vi "GUI_HTT_BeamNetUS_HOFI.vi"() -> ()   [LabVIEW 2020]
uses:
  Shared/GUI_Template/GUI_master/tcp_new_data_event.ctl
  Shared/GUI_Template/GUI_master/tcp new data cluster.ctl
  GUI_TestStand/Fire button.ctl
panel:
  in  "Tab Control 3":enum32{"Pointing"}(tab)
  in  "Position.Axis 321::20":dbl caption="HoleyMirror X" min=-9999999999.0 max=9999999999.0
  in  "Position.Axis 322::20":dbl caption="HoleyMirror Y" min=-999999.0 max=999999.0
  in  "Position.Axis 311::20":dbl caption="ScatterIn X" min=-999999.0 max=999999.0
  in  "Position.Axis 312::20":dbl caption="ScatterIn Y" min=-999999.0 max=999999.0
  in  "Front_BackScatter":bool
  out "ProbeToScatter (ns)":dbl format="%#_4g"
  out "Scatter Delay (ns)":dbl format="%#_4g"
  out "Probe Delay (ns)":dbl format="%#_4g"
  in  "value5::19":dbl caption="Drive t0 (P short)" min=-9999999.0 max=9999999.0 format="%#_13g"
  out "pressure::28":dbl caption="Measured\nPressure" min=-100.0 max=500.0 format="%#_13g"
  in  "GUIdevice 28":string="HTT-Baratron"
  in  "GUIdevice 27":string="HTT_LowPressureControl"
  in  "GUIdevice 26":string="HTT-HOFI_GasCellLength"
  in  "pressure::27":dbl caption="Set Pressure" min=0.0 max=500.0 format="%#_13g"
  in  "position::26":dbl caption="Length" min=0.0 max=104.0 format="%#_13g"
  in  "GUIdevice 25":string="HTT-Hexapod"
  out "ypos::25":dbl caption="ypos (longitudinal)" min=-22.0 max=22.0 format="%#_13g"
  out "zpos::25":dbl caption="zpos (vertical)" min=-10.0 max=10.0 format="%#_13g"
  in  "xpos::25":dbl caption="xpos (left/right)" min=-25.0 max=25.0 format="%#_13g"
  in  "Position.Axis 112::24":dbl caption="Scatter Comp. Y" min=-999999.0 max=999999.0
  in  "Position.Axis 111::24":dbl caption="Scatter Comp. X" min=-999999.0 max=999999.0
  in  "Position.Axis 522::24":dbl caption="TC_In_y" min=-999999.0 max=999999.0
  in  "Position.Axis 521::24":dbl caption="TC_In_x" min=-999999.0 max=999999.0
  in  "GUIdevice 19":string="HTT-Manual_Parameter"
  in  "value9::19":dbl caption="Scatter t0 (S)" min=-9999999.0 max=9999999.0 format="%#_13g"
  in  "value8::19":dbl caption="Scatter t0 (P long)" min=-9999999.0 max=9999999.0 format="%#_13g"
  in  "value6::19":dbl caption="Drive t0 (P long)" min=-9999999.0 max=9999999.0 format="%#_13g"
  in  "value7::19":dbl caption="Scatter t0 (P short)" min=-9999999.0 max=9999999.0 format="%#_13g"
  in  "Position.Axis 3::10":dbl caption="Drive Ghost Stage" min=0.0 max=50.0
  in  "Position.Axis 342::20":dbl caption="GhostY" min=-999999.0 max=999999.0
  in  "Position.Axis 341::20":dbl caption="GhostX" min=-999999.0 max=999999.0
  in  "Position.Axis 1::15":dbl caption="S stage" min=-600.0 max=600.0
  in  "position::23":dbl caption="P LongStage" min=0.0 max=610.0
  in  "Position.Axis 3::6":dbl caption="P ShortStage" min=0.0 max=200.0
  in  "GUIdevice 24":string="HTT-PicoPad_LCave"
  in  "Tab Control 2":enum32{"Longitudinal", "Transverse"}(tab)
  in  "Position.Axis 433::20":dbl caption="FFy (Chamber)" min=-999999.0 max=999999.0
  in  "Position.Axis 431::20":dbl caption="FFx (Chamber)" min=-999999.0 max=999999.0
  in  "Position.Axis 322::24":dbl caption="probe_y (L-Cave)" min=-999999.0 max=999999.0
  in  "Position.Axis 321::24":dbl caption="probe_x (L-Cave)" min=-999999.0 max=999999.0
  in  "Position.Axis 112::20":dbl caption="Probe_TC_InY" min=-999999.0 max=999999.0
  in  "Position.Axis 111::20":dbl caption="Probe_TC_InX" min=-999999.0 max=999999.0
  in  "GUIdevice 23":string="HTT_ProbeLongDelay"
  in  "GUIdevice 22":string="Assert-Ctrl_DUTStage"
  in  "GUIdevice 21":string="HTT-LPModeStage"
  in  "Position.Ch6::22":dbl caption="Back Ceramic" min=0.0 max=200.0
  in  "position::21":dbl caption="LP Mode Imager" min=0.0 max=400.0
  in  "Position.Axis 432::20":dbl caption="Axicon Pitch (y)" min=-999999.0 max=999999.0
  in  "Position.Axis 341::20":dbl caption="Axicon Yaw (x)" min=-999999.0 max=999999.0
  in  "Position.Axis 2::3":dbl caption="Axicon stage y" min=0.0 max=25.0
  in  "Position.Axis 1::3":dbl caption="Axicon stage x" min=0.0 max=25.0
  in  "Tab Control":enum32{"OAP", "Pointing"}(tab)
  in  "Position.Axis 142::20":dbl caption="OutY" min=-999999.0 max=999999.0
  in  "Position.Axis 141::20":dbl caption="OutX" min=-999999.0 max=999999.0
  in  "Position.Axis 132::20":dbl caption="OAPInY" min=-999999.0 max=999999.0
  in  "Position.Axis 131::20":dbl caption="OAPInX" min=-1e+19 max=9999999999999.0
  in  "Position.Axis 212::20":dbl caption="FFY" min=-999999.0 max=999999.0
  in  "Position.Axis 211::20":dbl caption="FFX" min=-999999.0 max=999999.0
  in  "Position.Axis 122::20":dbl caption="NFY" min=-999999.0 max=999999.0
  in  "Position.Axis 121::20":dbl caption="NFX" min=-999999.0 max=999999.0
  in  "GUIdevice 20":string="HTT-PicoPad_BCave"
  in  "GUIdevice 18":string="HTT-DG645_6_B"
  in  "GUIdevice 17":string="HTT-ManualParameterBool"
  in  "GUIdevice 16":string="HTT-DG645_5Hz"
  in  "GUIdevice 15":string="HTT-NewportXPS"
  out "fire::12":string="fire" caption="fire"
  in  "GUIdevice 14":string="HTT-Energy-S-G"
  in  "GUIdevice 13":string="HTT-Energy-D"
  in  "Position.Axis 2::11":dbl caption="Translation" min=-50.0 max=50.0
  in  "Position.Axis 3::11":dbl caption="Rotation G1" min=-360.0 max=360.0
  in  "Position.Axis 1::11":dbl caption="Rotation G2" min=-360.0 max=360.0
  in  "GUIdevice 12":string="HTT-DG645"
  out "Position.Axis3::2":dbl caption="Rotation G1" min=-180.0 max=180.0 format="%#_13g"
  out "Position.Axis2::2":dbl caption="Rotation G2" min=-180.0 max=180.0 format="%#_13g"
  in  "Position.Axis1::2":dbl caption="Translation" min=-60000.0 max=60000.0 format="%#_13g"
  in  "GUIdevice 11":string="HTT-ESP05"
  in  "GUIdevice 8":string="HTT-BNC"
  in  "GUIdevice 6":string="HTT-ESP04"
  in  "GUIdevice 5":string="HTT-ESP03"
  in  "Fire Button":T1=TRUE
  out "error IO 2":errorcluster
  out "fire::10":string
  out "tcp data event":T2
  in  "UDP error message":string
  in  "GUIdevice 7":string="HTT-Pulsar"
  in  "GUIdevice 2":string="HTT-Aerotech"
  in  "GUIdevice 10":string="HTT-ESP06"
  in  "GUIdevice 4":string="HTT-ESP02"
  in  "GUIdevice 1":string="HTT-MagTeslameter-DTM141"
  in  "GUIdevice 3":string="HTT-ESP01"
  in  "GUIdevice 9":string="HTT-HighPressureDAQ"
  in  "stop":bool
  # "Energy"
  # "CAP"
  # "BeamNetUS - HOFI"
  # "Drive"
  # "Probe"
  # "Pointing into TC"
  # "Alignment Stages"
  # "Target"
  # "Hexapod"
  # "Gas Cell"
  # "HOFI Compressor"
  # "HOFI line"
  # "Pointing into TC"
  # "Axicon"
  # "Timing"
  # "Drive Compressor"
  # "Stage Positions"
  # "Delays"
  # "Reference Measurements"
  # "v0.7   04/16/2021"
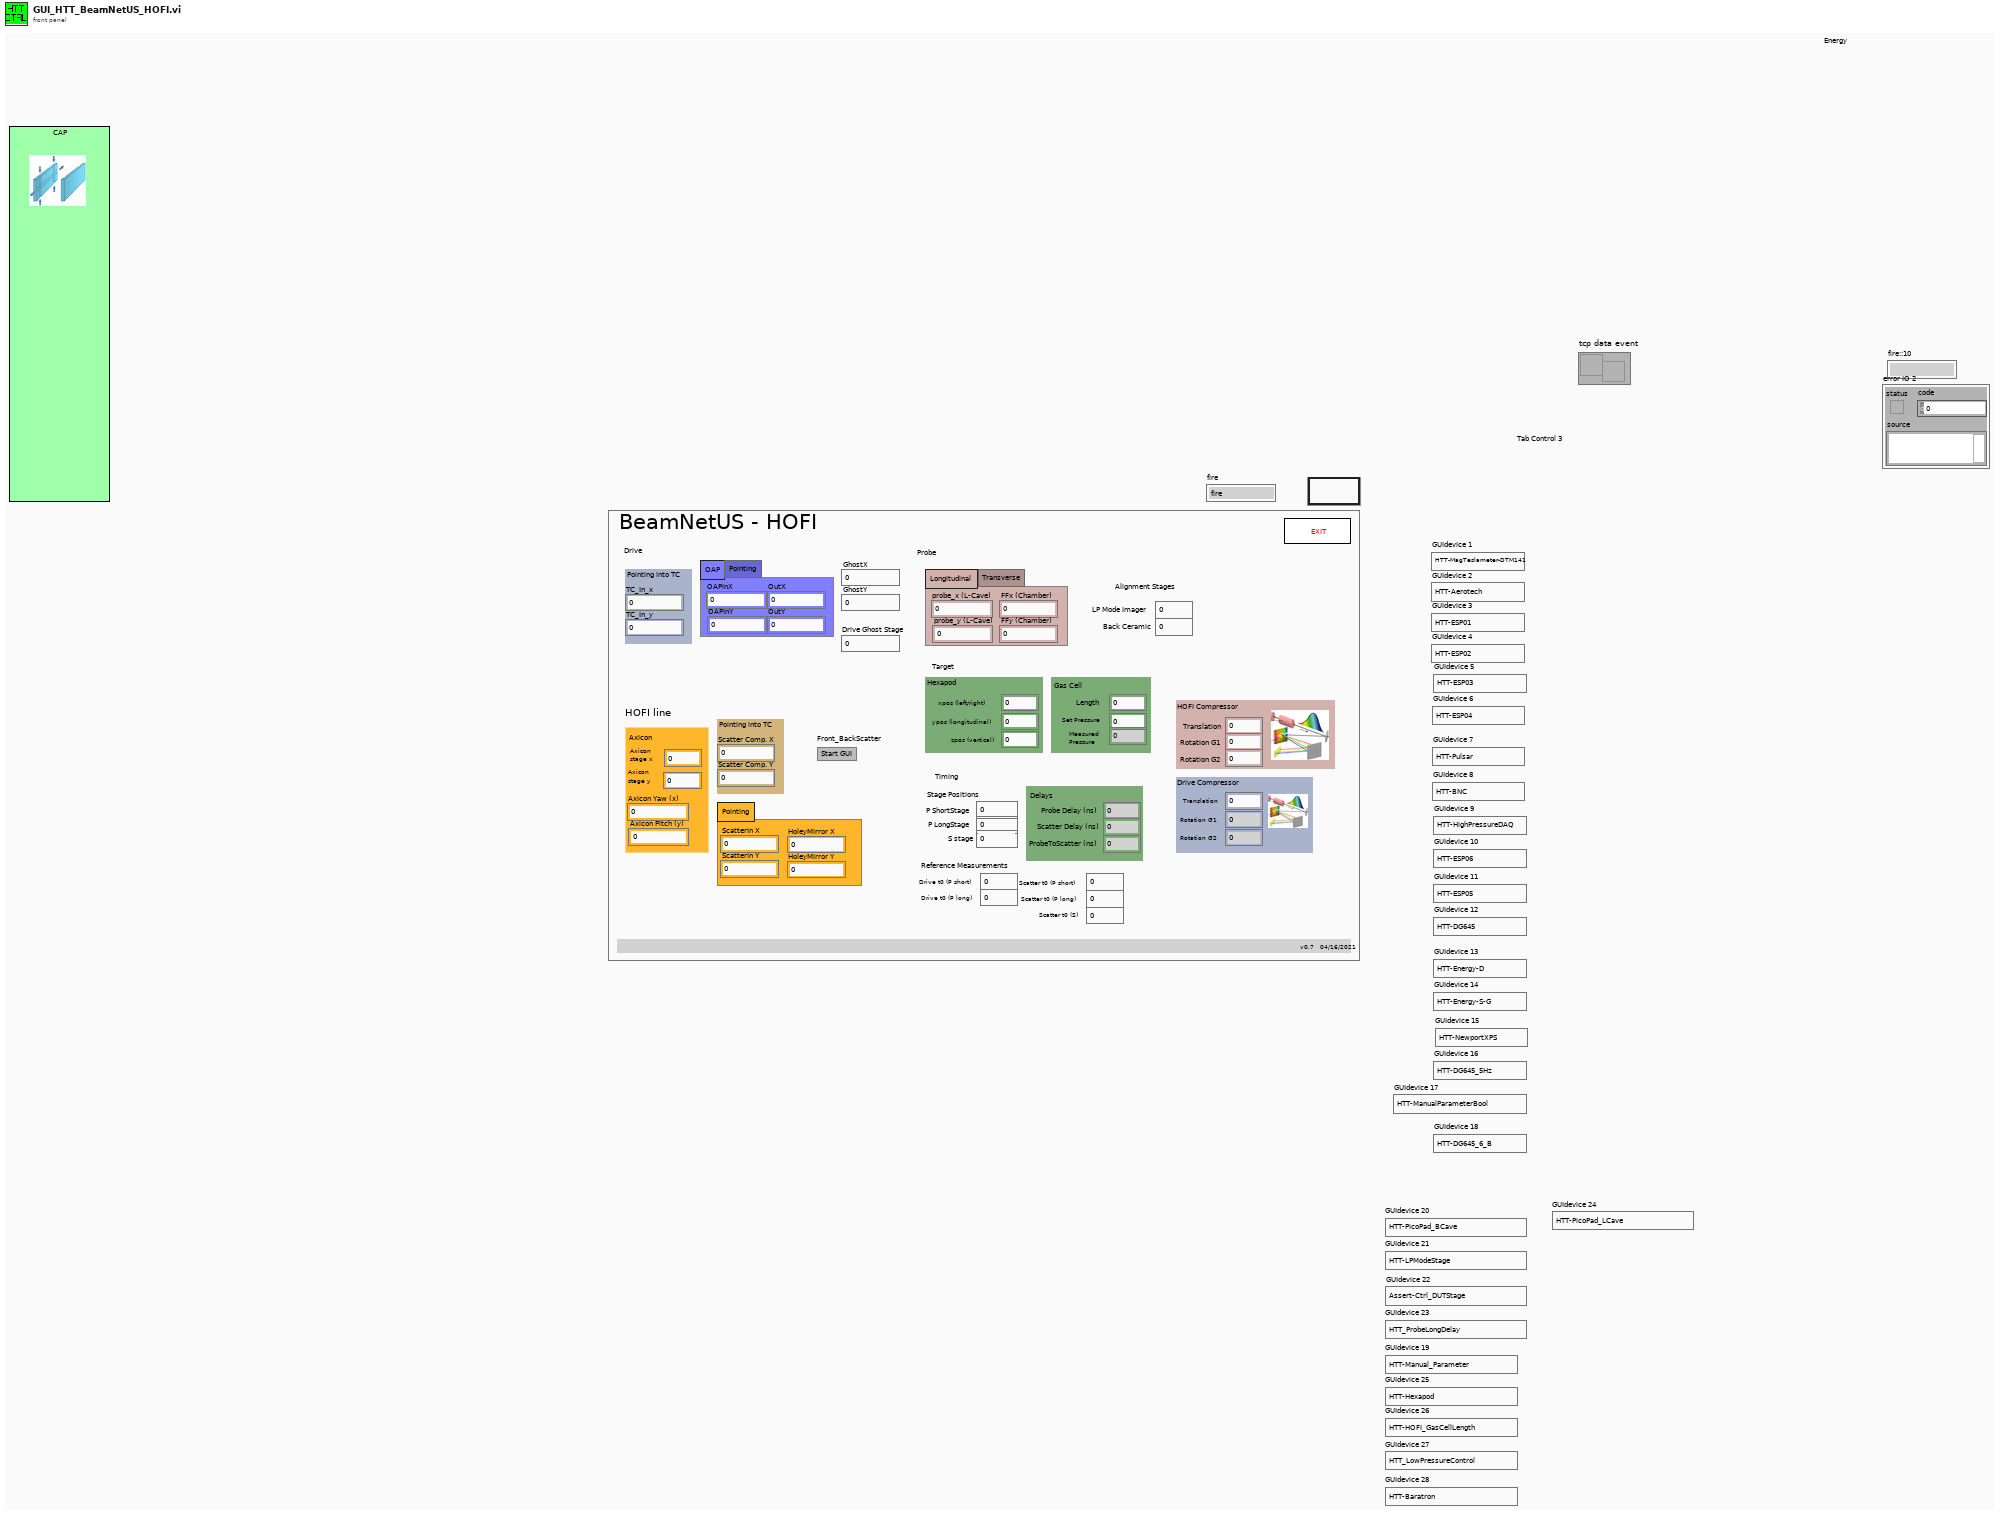
[diagram p1: front panel]
types:
  T1 = typedef "Fire button.ctl" = bool
  T2 = typedef "tcp_new_data_event.ctl" = refnum<user-event>
  T3 = typedef "tcp new data cluster.ctl" = cluster{"EventEnum":enum16{"new data", "connection status update"}, "Device name":string}
  T4 = enum32{"invalid app kind", "Development System", "Run Time System", "Student Edition", "Embedded LabVIEW", "Evaluation", "Custom"}
  T5 = enum32{"Invalid", "Standard", "Closed", "Hidden", "Minimized", "Maximized"}
  T6 = cluster{"Core":cluster{"Current VI Reference":refnum<vi>, "Close Panel on Exit?":bool}, "Heater timing offset":dbl, "Discharge timing offset":dbl, "Jet trigger":bool, "Tik1":u32, "Tik2":u32, "Fire Continues Allowed":bool, "Jet enable":bool}
  T7 = cluster{"Current VI Reference":refnum<vi>, "Close Panel on Exit?":bool}
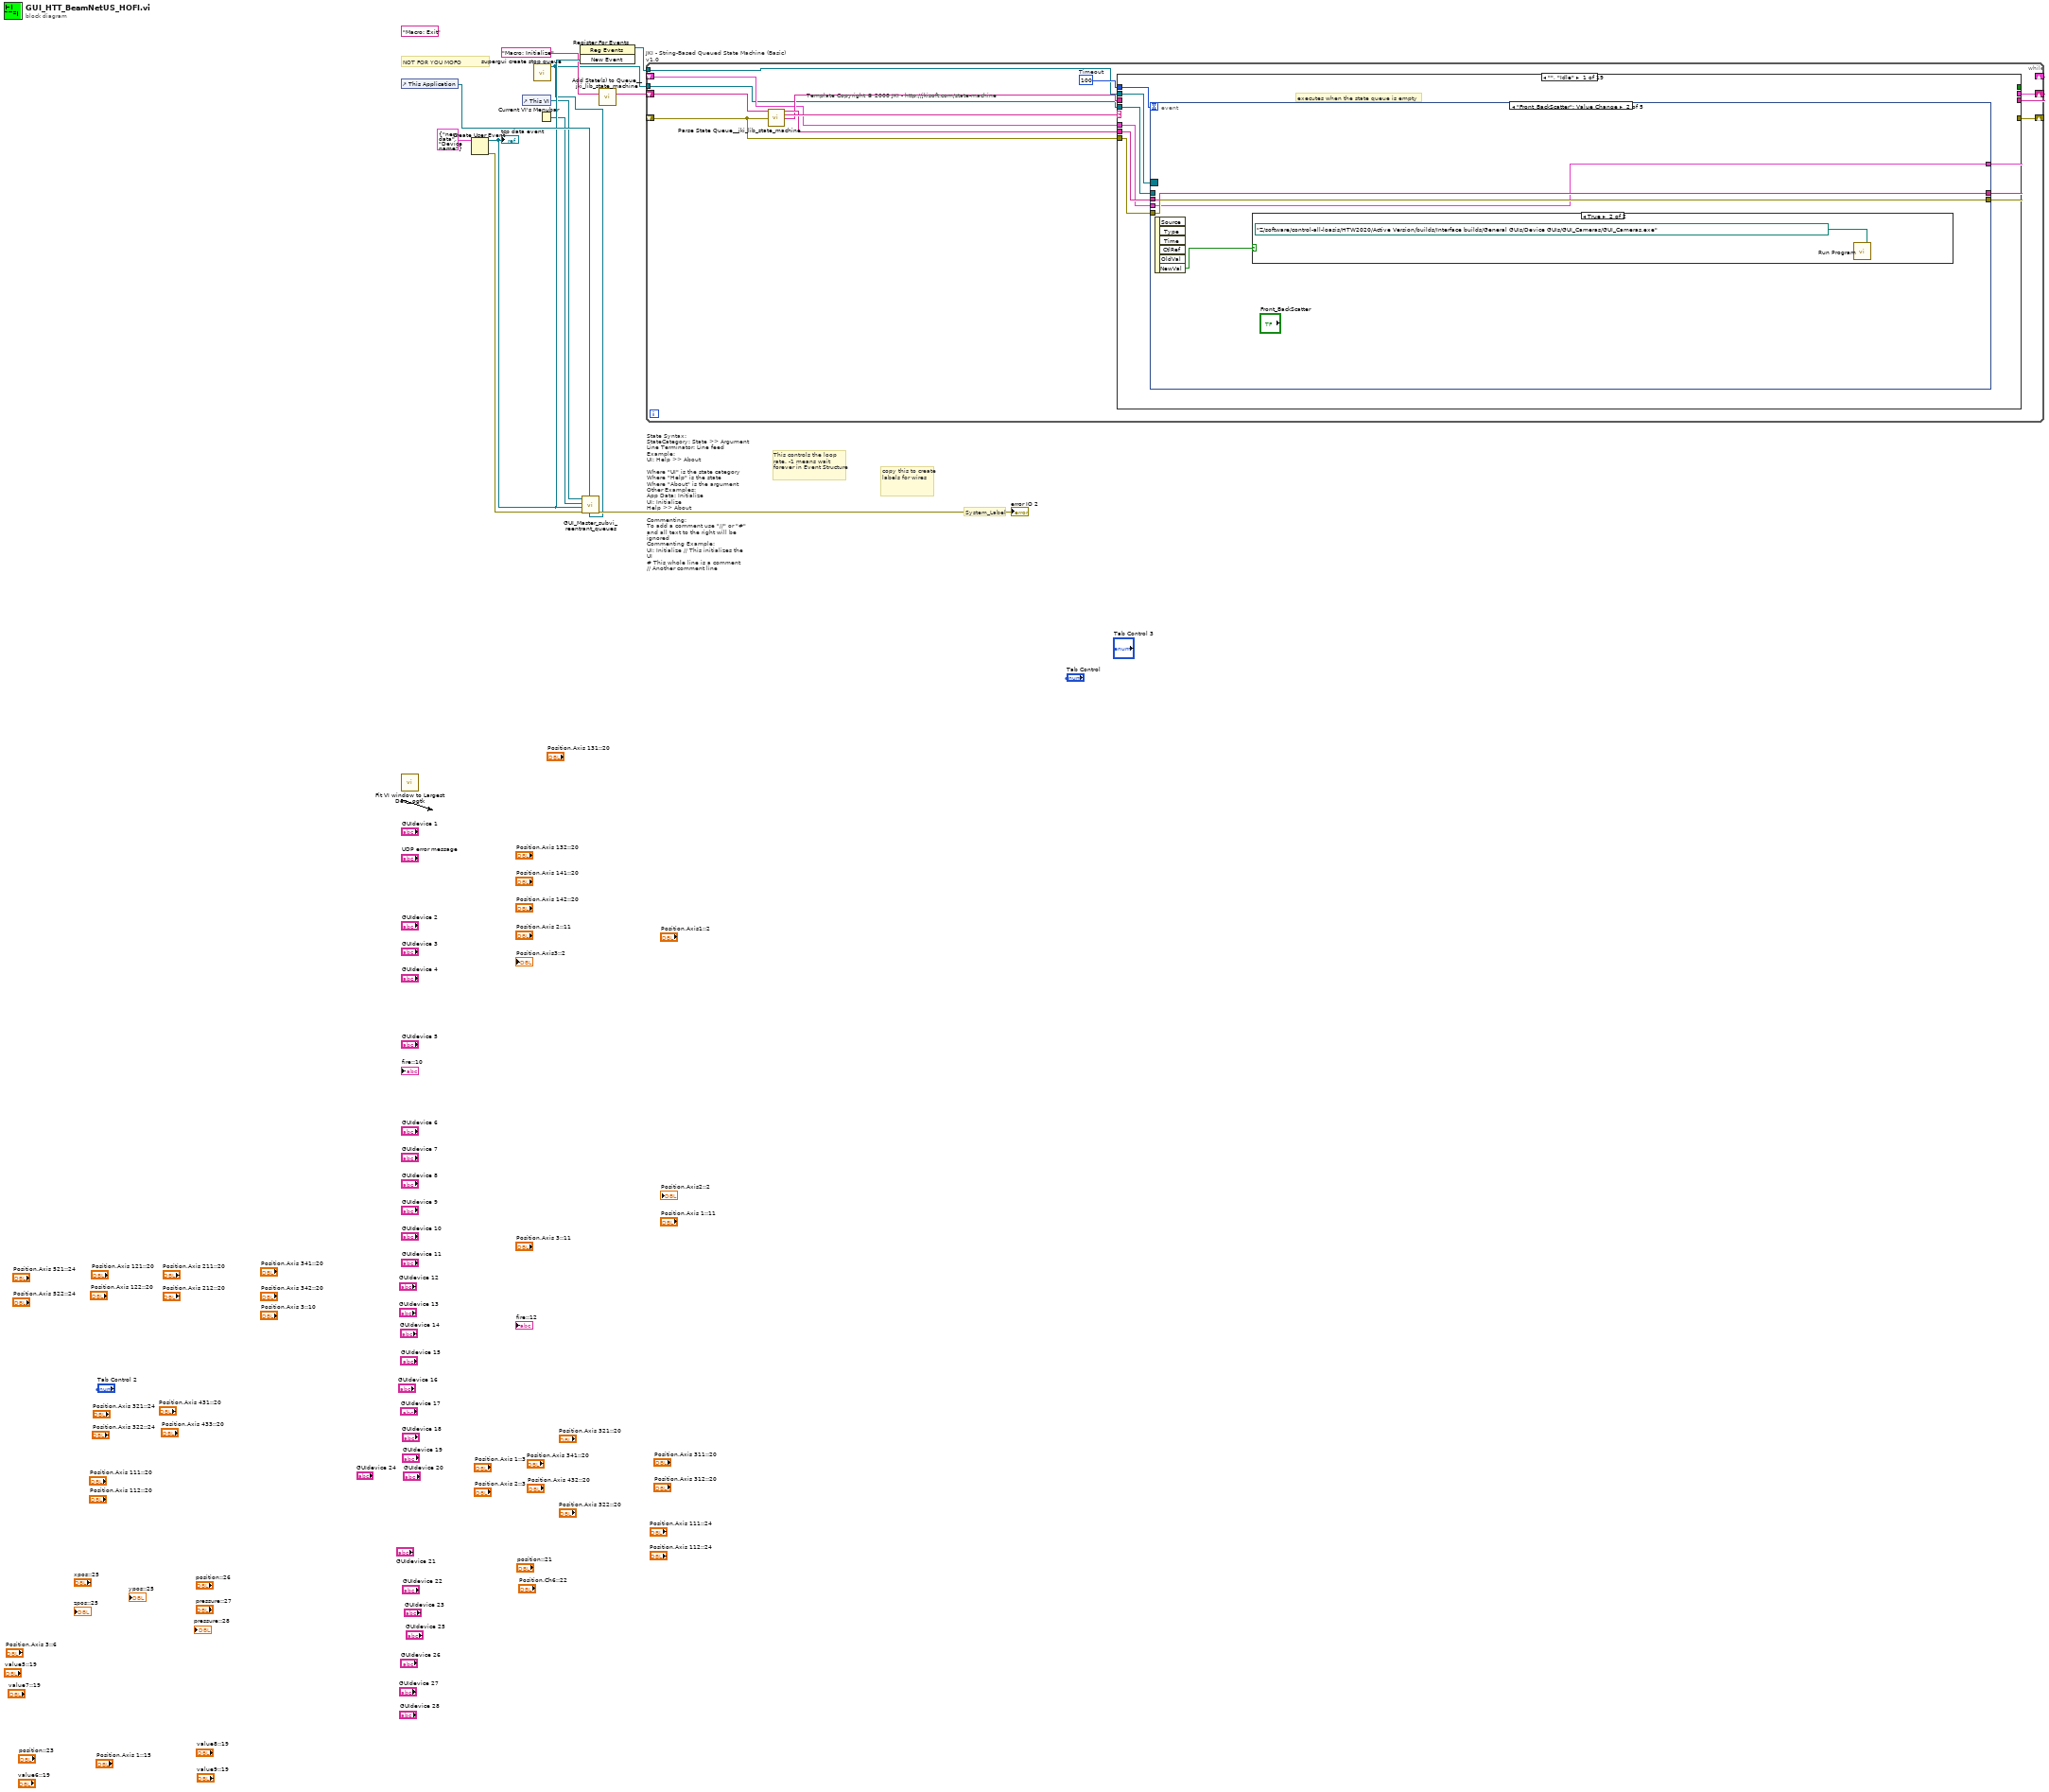
[diagram p0: block diagram]
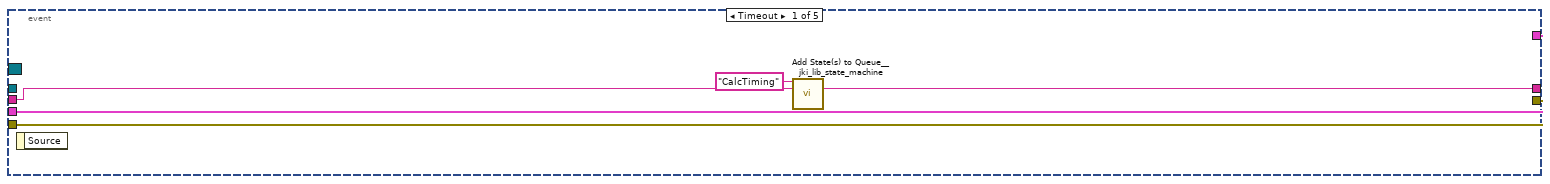
[diagram p2: hidden frame]
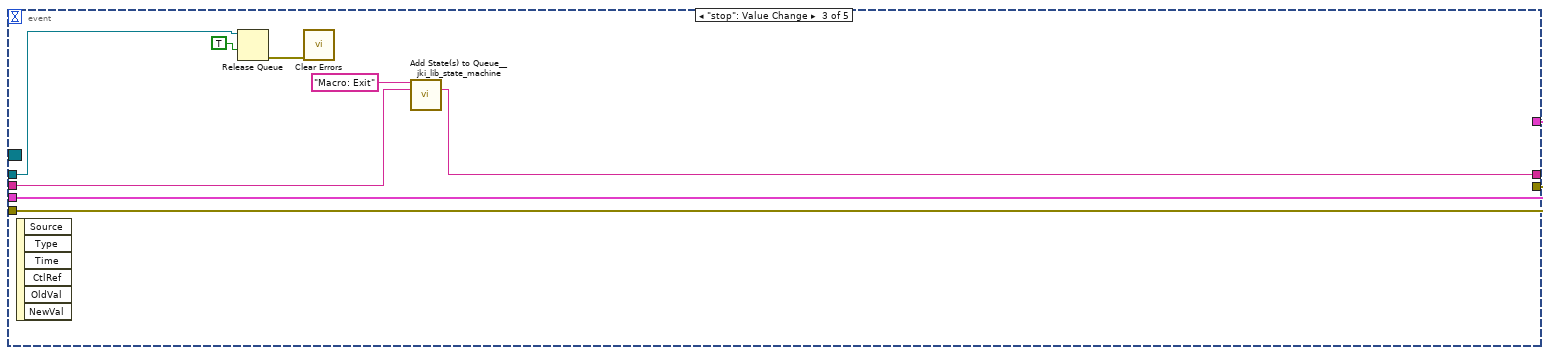
[diagram p4: hidden frame]
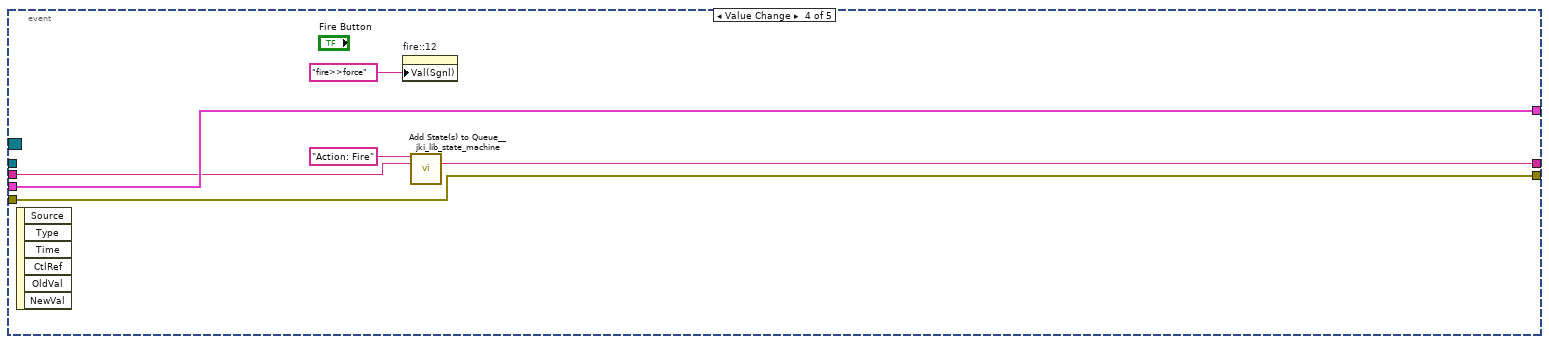
[diagram p5: hidden frame]
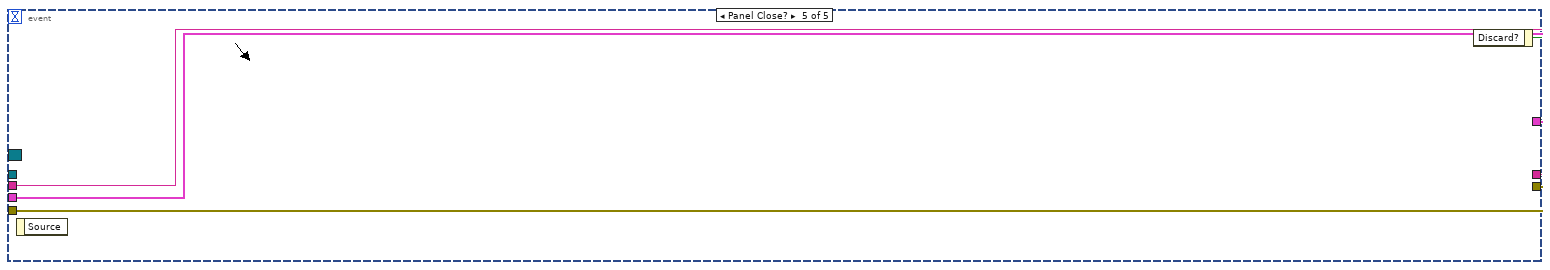
[diagram p6: hidden frame]
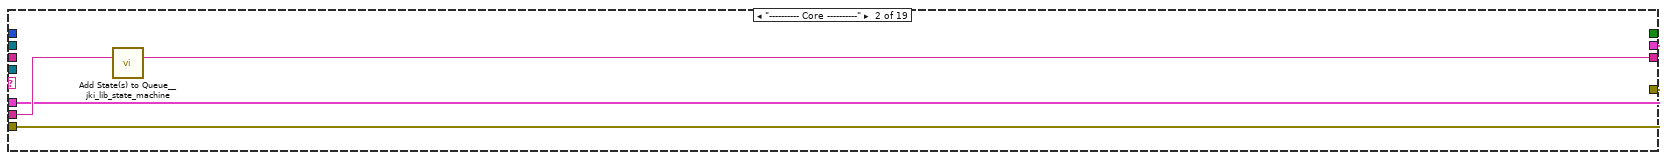
[diagram p7: hidden frame]
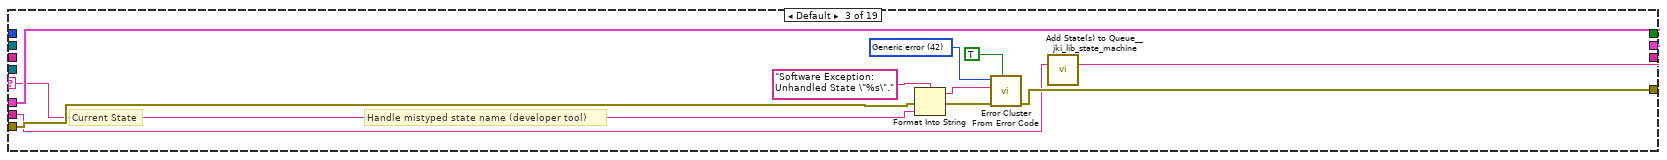
[diagram p8: hidden frame]
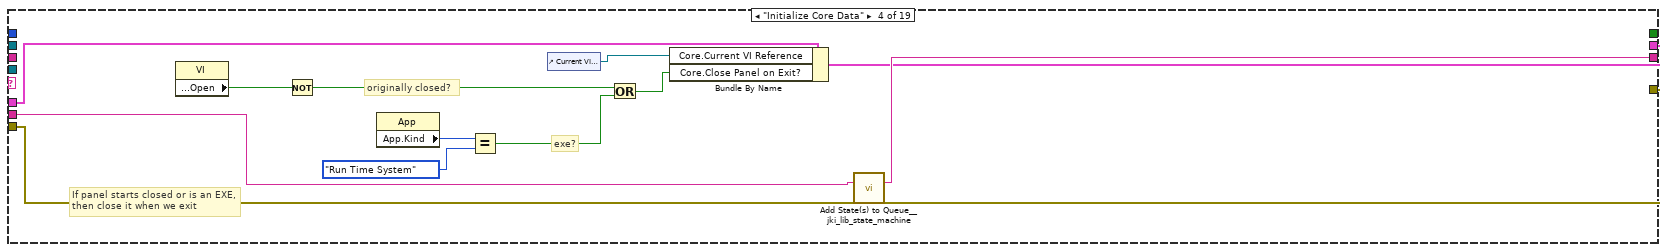
[diagram p9: hidden frame]
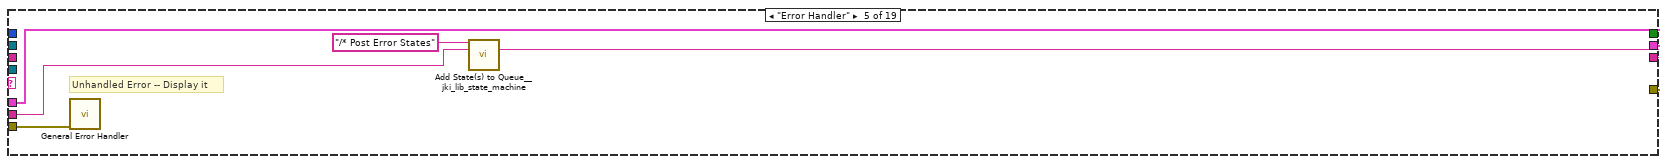
[diagram p10: hidden frame]
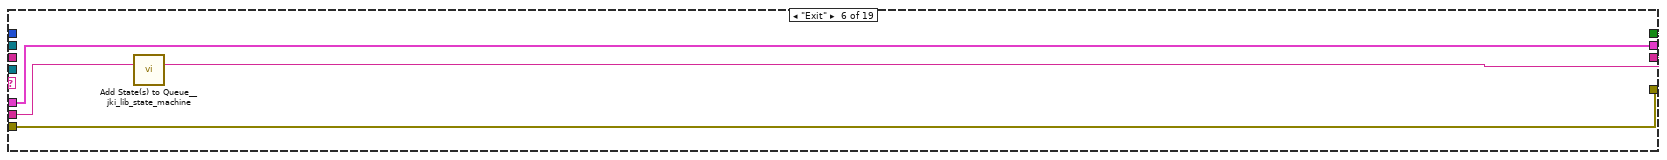
[diagram p11: hidden frame]
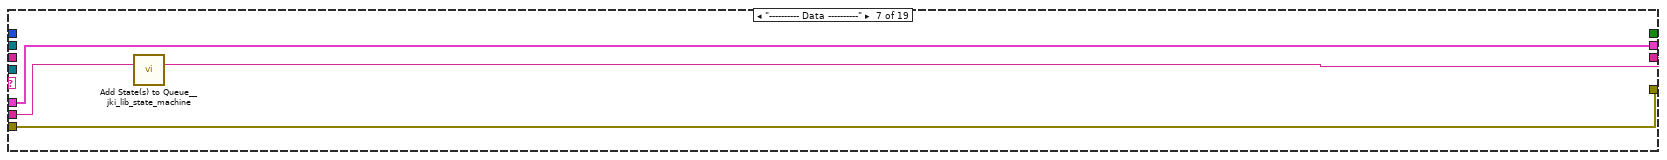
[diagram p12: hidden frame]
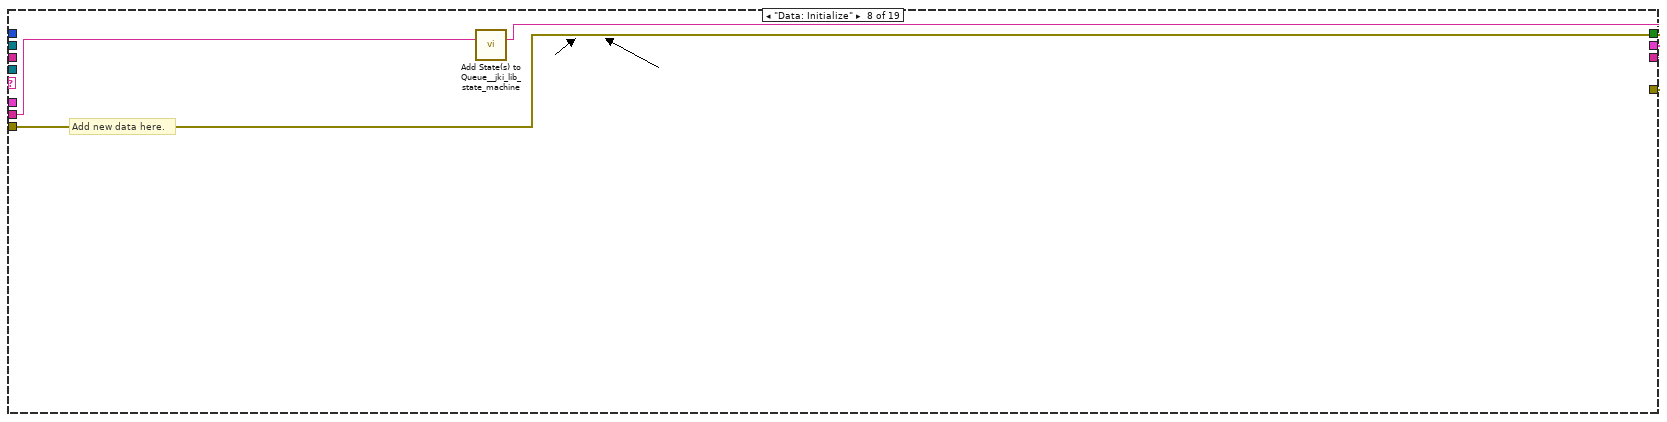
[diagram p13: hidden frame]
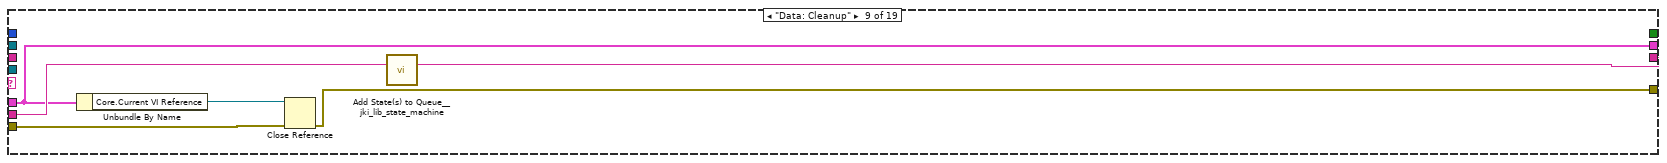
[diagram p14: hidden frame]
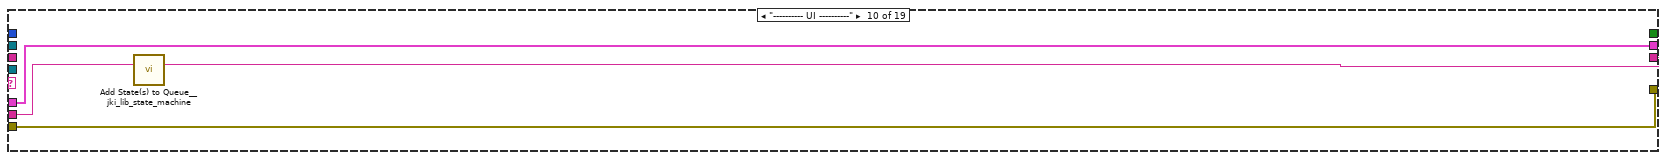
[diagram p15: hidden frame]
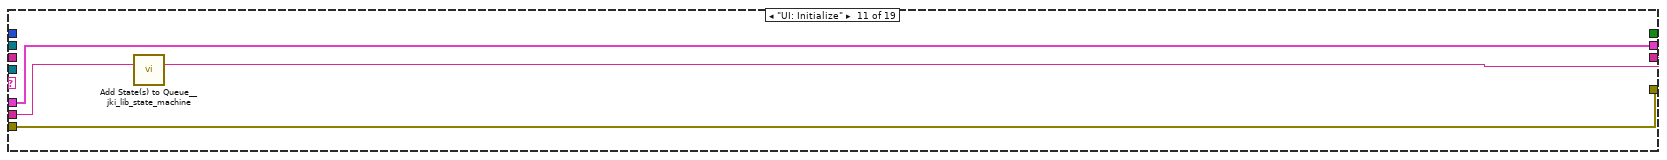
[diagram p16: hidden frame]
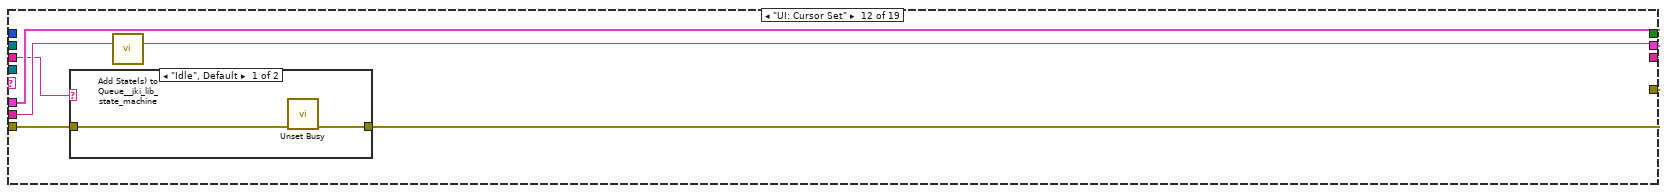
[diagram p17: hidden frame]
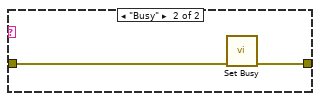
[diagram p18: hidden frame]
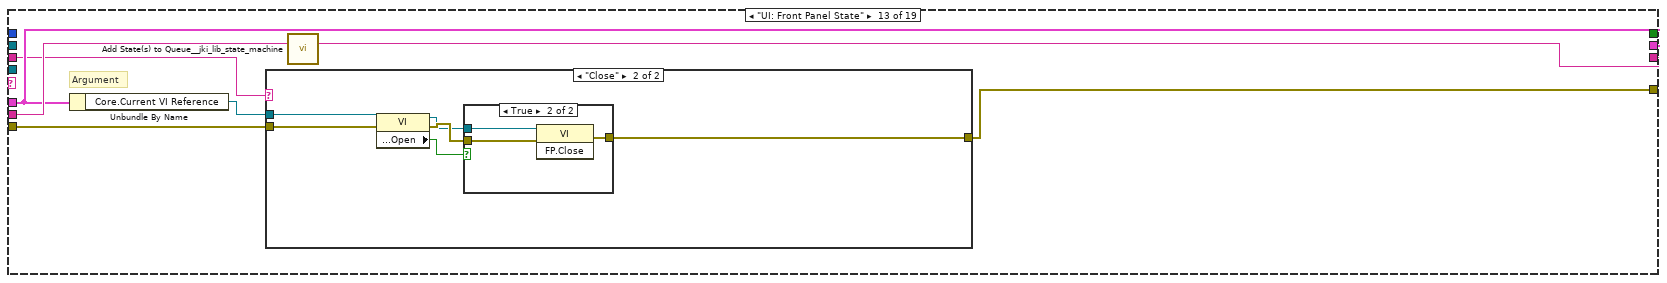
[diagram p19: hidden frame]
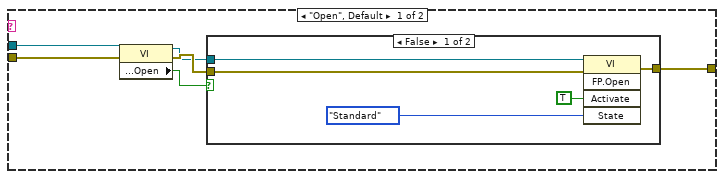
[diagram p20: hidden frame]
diagram:
  (unwired) "Macro: Exit"
  # "State Syntax:\nStateCategory: State >> Argument\nLine Terminator: Line feed\nExample:\nUI: Help >> About\n\nWhere \"UI\" is the state category\nWhere \"Help\" is the state\nWhere \"About\" is the argument\nOther Examples:\nApp Data: Initialize\nUI: Initialize\nHelp >> About\n\nCommenting:\nTo add a comment use \"//\" or \"#\" and all text to the right will be ignored\nCommenting Example:\nUI: Initialize // This initializes the UI\n# This whole line is a comment\n// Another comment line"
  # "copy this to create labels for wires"
  # "This controls the loop rate. -1 means wait forever in Event Structure"
  # "System_Label"
  # "NOT FOR YOU MOFO"
  n1 = control-ref of="This Application"() -> (w11:refnum<vi>)
  n2 = call <userlib>:"Fit VI window to Largest Dec__ogtk.vi"() -> ()  [unwired: 6 in, 2 out]
  n3 = Create User Event(user event datatype=T3 {"EventEnum"=enum."new data", "Device name"="Device name"} ("New Event")) -> (user event=w10:refnum<user-event>, error out=w9:errorcluster)  [unwired: 1 in]
  "tcp data event" <- w10
  n4 = control-ref of="This VI"() -> (w5:refnum<vi>)
  n5 = call "supergui create stop queue.vi"() -> ("STOP Queue out"=w2:refnum<queue>)  [unwired: 11 in]
  n6 = Current VI's Menubar() -> (w7:refnum<k9>)
  n7 = register-events(w10) -> (reference out=w1:refnum<event-registration>)  [unwired: 2 in, 1 out]
  n8 = call "GUI_Master_subvi_reentrant_queues.vi"("STOP Queue in"=w2, "This Application"=w11, "error in (no error)"=w9, "tcp data event"=w10, "Caller menu reference"=w7, "Caller VI ref"=w5) -> ("error out"=→"error IO 2":errorcluster)  [unwired: 5 in]
  n9 = call <vilib>:"Add State(s) to Queue__jki_lib_state_machine.vi"("State(s) in (\"\")"="Macro: Initialize") -> ("States Out"=w3:string)  [unwired: 14 in]
  n10 = while "JKI - String-Based Queued State Machine (Basic) v1.0" {
    shift-right: [w18] -> _
    shift-left: _ -> [w17]
    shift-right: [w20] -> _
    shift-left: _ -> [w15]
    shift-right: [w19] -> _
    shift-left: w3 -> [w21]
    tunnel: w1 -> [w14]
    tunnel: w2 -> [w13]
    stop <- w12 stop-if-true
    w16 = 100  # Timeout
    # "Template Copyright © 2008 JKI - http://jkisoft.com/state-machine"
    n11 = call <vilib>:"Parse State Queue__jki_lib_state_machine.vi"("State Queue"=w21, "Error In (no error)"=w15) -> ("Remaining States"=w23:string, "Current State"=w24:string, "Arguments"=w22:string)  [unwired: 11 in]
    n12 = case shown="\"\", \"Idle\"" w24 {
      selector: w24 -> [_ _ w68 _ _ _ _ _ _ _ _ _ _ _ _ _ _ _ _]
      tunnel: w23 -> [w33 w67 w72 w90 w96 w101 w105 w117 w123 w127 w131 w137 w148 w174 w211 w216 w226 w230 w236]
      tunnel: w22 -> [_ _ _ _ _ _ _ _ _ _ _ w132 w142 _ _ _ _ _ _]
      tunnel: w17 -> [w31 w64 w70 w81 w93 w99 w102 _ w118 w124 w129 w135 w144 w171 w208 w213 w223 w227 w234]
      tunnel: [w30 w65 w74 w87 errorcluster {"status"=FALSE, "code"=0, "source"=""} ("error out") w98 w103 w114 w119 w125 w128 w133 w145 w172 w209 w214 w224 w228 w231] -> w20
      tunnel: w15 -> [w29 w65 w73 w87 w92 w98 w103 w114 w120 w125 w128 w134 w146 w172 w209 w214 w224 w228 w232]
      tunnel: [w32 w66 w71 w89 w95 w100 w104 w116 w122 w126 w130 w136 w147 w173 w210 w215 w225 w229 w235] -> w19
      tunnel: [_ _ _ _ _ TRUE _ _ _ _ _ _ _ _ _ _ _ _ _] -> w12
      tunnel: [w25 w64 w70 w88 w93 w99 w102 w115 w118 w124 w129 w135 w144 w171 w208 w213 w223 w227 w234] -> w18
      tunnel: w16 -> [w28 _ _ _ _ _ _ _ _ _ _ _ _ _ _ _ _ _ _]
      tunnel: w14 -> [w27 _ _ _ _ _ _ _ _ _ _ _ _ _ _ _ _ _ _]
      tunnel: w13 -> [w26 _ _ _ _ _ _ _ _ _ _ _ _ _ _ _ _ _ _]
      frame "", "Idle" {
        # "executes when the state queue is empty"
        n13 = event shown="[1] \"Front_BackScatter\": Value Change" {
          selector: w27 -> [_ _ _ _ _]
          dyn-events: _ -> [_ _ _ _ _]
          timeout: w28 -> [_ _ _ _ _]
          tunnel: w33 -> [w38 w40 w51 w54 w63]
          tunnel: [w37 w40 w50 w55 w62] -> w32
          tunnel: w31 -> [w35 w39 w48 w57 w60]
          tunnel: [w36 w41 w49 w56 w61] -> w30
          tunnel: w29 -> [w36 w41 w49 w56 w61]
          tunnel: [w35 w39 w48 w57 w60] -> w25
          tunnel: w26 -> [_ _ w45 _ _]
          event Timeout {
            n14 = event-data() -> ()  [unwired: 1 in, 1 out]
            n15 = call <vilib>:"Add State(s) to Queue__jki_lib_state_machine.vi"("State(s) in Front (\"\")"="CalcTiming" ("State(s) in Front (\"\")"), "State(s) in (\"\")"=w38) -> ("States Out"=w37:string)  [unwired: 13 in]
          }
          event "Front_BackScatter": Value Change {
            n16 = event-data() -> ("NewVal"=w42:bool)  [unwired: 1 in, 5 out]
            n17 = case shown="True" w42 {
              frame False {
              }
              frame True {
                n18 = call "Run Program.vi"("Program Path"=path "Z:/software/control-all-loasis/HTW2020/Active Version/builds/Interface builds/General GUIs/Device GUIs/GUI_Cameras/GUI_Cameras.exe") -> ()  [unwired: 1 in]
              }
            }
          }
          event "stop": Value Change {
            # "Exit Button Value Change (pressed) Event\n(this executes Macro: Exit to terminate the VI)"
            n19 = event-data() -> ()  [unwired: 1 in, 6 out]
            n20 = Release Queue(queue=w45, force destroy? (F)=TRUE) -> (error out=w46:errorcluster)  [unwired: 1 in, 2 out]
            n21 = call <vilib>:"Clear Errors.vi"("error in (no error)"=w46) -> ()  [unwired: 5 in, 2 out]
            n22 = call <vilib>:"Add State(s) to Queue__jki_lib_state_machine.vi"("State(s) in Front (\"\")"="Macro: Exit", "State(s) in (\"\")"=w51) -> ("States Out"=w50:string)  [unwired: 13 in]
          }
          event Value Change {
            n23 = event-data() -> ()  [unwired: 1 in, 6 out]
            n24 = property on="fire::12" class="Str"("Val(Sgnl)"="fire>>force" ("Value (Signaling)")) -> ()  [unwired: 2 in, 2 out]
            n25 = call <vilib>:"Add State(s) to Queue__jki_lib_state_machine.vi"("State(s) in Front (\"\")"="Action: Fire" ("State(s) in Front (\"\")"), "State(s) in (\"\")"=w54) -> ("States Out"=w55:string)  [unwired: 13 in]
          }
          event Panel Close? {
            # "Discard the event because we'll close the front panel ourselves in Macro: Exit"
            # "Close Panel button (pressed) Event\n(this executes Macro: Exit to terminate the VI)"
            n26 = event-data() -> ()  [unwired: 1 in, 1 out]
            n27 = event-data("Discard?"=TRUE) -> ()  [unwired: 1 in, 1 out]
            n28 = call <vilib>:"Add State(s) to Queue__jki_lib_state_machine.vi"("State(s) in Front (\"\")"="Macro: Exit", "State(s) in (\"\")"=w63) -> ("States Out"=w62:string)  [unwired: 13 in]
          }
        }
      }
      frame "---------- Core ----------" {
        # "Do not put any code in this frame.\n(it is a separator no-op)"
        n29 = call <vilib>:"Add State(s) to Queue__jki_lib_state_machine.vi"("State(s) in (\"\")"=w67) -> ("States Out"=w66:string)  [unwired: 14 in]
      }
      frame Default {
        w77 = 42 items=["No error", "Argument error", "Memory is full", "Out of zone", "End of file", "File already open", "Generic file I/O error", "File not found", "File permission error", "Disk is full", "Duplicate path", "Too many files open", "System feature not enabled", "Resource file not found", "Cannot add resource", "Resource not found", "Image not found", "Image memory error", "Pen does not exist", "Config type invalid", "Config token not found", "Config parse error", "Config memory error", "Bad external code format", "Bad external code offset", "External code not present", "Null window", "Destroy window error", "Null menu", "Print aborted", "Bad print record", "Print driver error", "Windows error during printing", "Memory error during printing", "Print dialog error", "Generic print error", "Invalid device refnum", "Device not found", "Device parameter error", "Device unit error", "Cannot open device", "Device call aborted", "Generic error", "Cancelled by user", "Object ID too low", "Object ID too high", "Object not in heap", "Unknown heap", "Unknown object (invalid DefProc)", "Unknown object (DefProc not in table)", "Message out of range", "Invalid (null) method", "Unknown message", "Manager call not supported", "Bad address", "Network operation in progress", "Network operation timed out", "Connection is busy", "Network attribute not supported", "Network error", "Address in use", "System out of memory", "Connection aborted", "Connection refused", "Not connected", "Already connected", "Connection closed", "Initialization error (interapplication manager)", "Bad occurrence", "Wait on unbound occurrence handler", "Occurrence queue overflow", "Datalog type conflict", "Unused", "Unrecognized type (interapplication manager)", "Memory corrupt", "Failed to make temporary DLL", "Old CIN version", "Drag socket not found", "Failed to load drop-object", "Failed to register OLE object", "Failed to release OLE object", "Format specifier type mismatch", "Unknown format specifier", "Too few format specifiers", "Too many format specifiers", "Scan failed", "Newer CIN version", "Error converting to variant", "Runtime menu error", "Password tampered", "Variant attribute not found", "Incompatible variant data type", "Event data is not available", "Event Store is not present", "Occurrence is not found", "Event Queue is not created", "Event info is not available", "Refnum passed is NULL", "Error retrieving Class GUID", "Error retrieving CoClass GUID", "Error retrieving TypeLib GUID.", "Bad built application magic bytes.", "Specific driver is different from the specific driver associated with the Logical Name.", "There is no session opened to the class driver.", "Max Error", "MAX - Error with config objects", "MAX - Error loading configuration", "MAX - Group not supported"]
        # "Current State"
        # "Do not delete, rename, or modify this frame.\n(this is used to capture unhandled states and typos)"
        # "Handle mistyped state name (developer tool)"
        n30 = Format Into String(format string="Software Exception: Unhandled State \"%s\"." ("message"), error in=w73, w68) -> (resulting string=w76:string, error out=w75:errorcluster)  [unwired: 1 in]
        n31 = call <vilib>:"Error Cluster From Error Code.vi"("show call chain? (False)"=TRUE, "error in (no error)"=w75, "error message (\"\")"=w76, "error code (0)"=w77) -> ("error out"=w74:errorcluster)  [unwired: 5 in]
        n32 = call <vilib>:"Add State(s) to Queue__jki_lib_state_machine.vi"("State(s) in (\"\")"=w72) -> ("States Out"=w71:string)  [unwired: 14 in]
      }
      frame "Initialize Core Data" {
        # "Do not delete, rename, or modify this frame.\n(this is used to determine panel behavior on exit)"
        # "originally closed?"
        # "exe?"
        # "If panel starts closed or is an EXE, then close it when we exit"
        n33 = property class="VI"() -> ("Front Panel.Open"=w86:bool)  [unwired: 2 in, 2 out]
        n34 = Not(x=w86) -> (.not. x?=w83:bool)
        n35 = property class="App"() -> ("App.Kind"=w85:T4)  [unwired: 2 in, 2 out]
        n36 = Equal?(x=w85, y=T4."Run Time System" ("Application:Kind")) -> (x = y?=w82:bool)
        n37 = control-ref of="Current VI Reference"() -> (w79:refnum<vi>)
        n38 = Or(x=w83, y=w82) -> (x .or. y?=w80:bool)
        n39 = Bundle By Name(cluster=w81, "Core.Current VI Reference"=w79, "Core.Close Panel on Exit?"=w80) -> (w88:T6)
        n40 = call <vilib>:"Add State(s) to Queue__jki_lib_state_machine.vi"("State(s) in (\"\")"=w90) -> ("States Out"=w89:string)  [unwired: 14 in]
      }
      frame "Error Handler" {
        # "Unhandled Error -- Display it"
        # "Handle any errors here.\nYou can also output any states to clean-up after errors occur"
        # "Clear error"
        n41 = call <vilib>:"General Error Handler.vi"("error in (no error)"=w92) -> ()  [unwired: 10 in, 5 out]
        n42 = call <vilib>:"Add State(s) to Queue__jki_lib_state_machine.vi"("State(s) in Front (\"\")"="/* Post Error States", "State(s) in (\"\")"=w96) -> ("States Out"=w95:string)  [unwired: 13 in]
      }
      frame "Exit" {
        # "Do not put any code in this frame.\n(No errors that occur here will be handled.)"
        n43 = call <vilib>:"Add State(s) to Queue__jki_lib_state_machine.vi"("State(s) in (\"\")"=w101) -> ("States Out"=w100:string)  [unwired: 14 in]
      }
      frame "---------- Data ----------" {
        # "Do not put any code in this frame.\n(It is a separator no-op. You can make a copy of this frame to create a new Data frame)"
        n44 = call <vilib>:"Add State(s) to Queue__jki_lib_state_machine.vi"("State(s) in (\"\")"=w105) -> ("States Out"=w104:string)  [unwired: 14 in]
      }
      frame "Data: Initialize" {
        w106 = FALSE  # Jet enable
        w107 = FALSE  # Fire Continues Allowed
        w109 = u32 0  # Tik1
        w108 = u32 0  # Tik2
        w110 = FALSE  # Jet trigger
        w111 = 0.0  # Discharge timing offset
        w112 = 0.0  # Heater timing offset
        w113 = T7 {"Current VI Reference"=refnum, "Close Panel on Exit?"=FALSE}  # Core
        # "do not delete - used by framework"
        # "Expand Bundle to add new data elements to shift register data."
        # "Add new data here."
        # "Data names and types of shift register data are defined by this bundle."
        # "Initialize the shift-register data, here.\n(data names are defined by what you wire into the bundle function)"
        n45 = call <vilib>:"Add State(s) to Queue__jki_lib_state_machine.vi"("State(s) in (\"\")"=w117) -> ("States Out"=w116:string)  [unwired: 14 in]
        n46 = Bundle("Core"=w113, "Heater timing offset"=w112, "Discharge timing offset"=w111, "Jet trigger"=w110, "Tik1"=w109, "Tik2"=w108, "Fire Continues Allowed"=w107, "Jet enable"=w106) -> (w115:T6)  [unwired: 1 in]
      }
      frame "Data: Cleanup" {
        # "Cleanup any data and references, here.\n(this is called automatically, by the Macro: Exit)"
        n47 = Unbundle By Name(w118) -> ("Core.Current VI Reference"=w121:refnum<vi>)
        n48 = Close Reference(reference=w121, error in (no error)=w120) -> (error out=w119:errorcluster)
        n49 = call <vilib>:"Add State(s) to Queue__jki_lib_state_machine.vi"("State(s) in (\"\")"=w123) -> ("States Out"=w122:string)  [unwired: 14 in]
      }
      frame "---------- UI ----------" {
        # "Do not put any code in this frame.\n(It is a separator no-op. You can make a copy of this frame to create a new UI frame)"
        n50 = call <vilib>:"Add State(s) to Queue__jki_lib_state_machine.vi"("State(s) in (\"\")"=w127) -> ("States Out"=w126:string)  [unwired: 14 in]
      }
      frame "UI: Initialize" {
        # "Initialize the User Interface, here.\n(this is called automatically, by the Macro: Init)"
        n51 = call <vilib>:"Add State(s) to Queue__jki_lib_state_machine.vi"("State(s) in (\"\")"=w131) -> ("States Out"=w130:string)  [unwired: 14 in]
      }
      frame "UI: Cursor Set" {
        # "Argument"
        # "Set and Unset Cursor Busy.\n(Usage: \"UI: Cursor Set >> Busy|Idle\")"
        n52 = case shown="\"Idle\", Default" w132 {
          tunnel: w134 -> [w139 w141]
          tunnel: [w138 w140] -> w133
          frame "Idle", Default {
            n53 = call <vilib>:"Unset Busy.vi"("error in (no error)"=w139) -> ("error out"=w138:errorcluster)  [unwired: 10 in]
          }
          frame "Busy" {
            n54 = call <vilib>:"Set Busy.vi"("error in (no error)"=w141) -> ("error out"=w140:errorcluster)  [unwired: 9 in, 1 out]
          }
        }
        n55 = call <vilib>:"Add State(s) to Queue__jki_lib_state_machine.vi"("State(s) in (\"\")"=w137) -> ("States Out"=w136:string)  [unwired: 14 in]
      }
      frame "UI: Front Panel State" {
        # "Argument"
        # "Set Front Panel Open or Closed\n(Usage: \"UI: Front Panel State >> Open|Close\")"
        n56 = Unbundle By Name(w144) -> ("Core.Current VI Reference"=w143:refnum<vi>)
        n57 = case shown="\"Close\"" w142 {
          tunnel: w146 -> [w152 w165]
          tunnel: [w154 w166] -> w145
          tunnel: w143 -> [w153 w163]
          frame "Open", Default {
            n58 = property class="VI"(reference=w153, error in=w152) -> (reference out=w150:refnum<vi>, error out=w151:errorcluster, "Front Panel.Open"=w149:bool)
            n59 = case shown="False" w149 {
              tunnel: [w157 w160] -> w154
              tunnel: w151 -> [w156 w160]
              tunnel: w150 -> [w155 _]
              frame False {
                n60 = invoke class="VI" method="FP.Open"(reference=w155, error in=w156, "Activate"=TRUE, "State"=T5."Standard") -> (error out=w157:errorcluster)  [unwired: 1 in, 4 out]
              }
              frame True {
              }
            }
          }
          frame "Close" {
            n61 = property class="VI"(reference=w163, error in=w165) -> (reference out=w162:refnum<vi>, error out=w164:errorcluster, "Front Panel.Open"=w161:bool)
            n62 = case shown="True" w161 {
              tunnel: [w167 w170] -> w166
              tunnel: w164 -> [w167 w169]
              tunnel: w162 -> [_ w168]
              frame False {
              }
              frame True {
                n63 = invoke class="VI" method="FP.Close"(reference=w168, error in=w169) -> (error out=w170:errorcluster)  [unwired: 1 in, 2 out]
              }
            }
          }
        }
        n64 = call <vilib>:"Add State(s) to Queue__jki_lib_state_machine.vi"("State(s) in (\"\")"=w148) -> ("States Out"=w147:string)  [unwired: 14 in]
      }
      frame "---------- Macro ----------" {
        # "Do not put any code in this frame.\n(It is a separator no-op. You can make a copy of this frame to create a new Macro frame)"
        n65 = call <vilib>:"Add State(s) to Queue__jki_lib_state_machine.vi"("State(s) in (\"\")"=w174) -> ("States Out"=w173:string)  [unwired: 14 in]
      }
      frame "CalcTiming" {
        # "Do not put any code in this frame.\n(It is a separator no-op. You can make a copy of this frame to create a new Macro frame)"
        n66 = property on="value7::19" class="DigNum (strict)"() -> ("Value"=w182:dbl)  [unwired: 2 in, 2 out]
        n67 = property on="value5::19" class="DigNum (strict)"() -> ("Value"=w183:dbl)  [unwired: 2 in, 2 out]
        n68 = property on="value8::19" class="DigNum (strict)"() -> ("Value"=w188:dbl)  [unwired: 2 in, 2 out]
        n69 = property on="value6::19" class="DigNum (strict)"() -> ("Value"=w187:dbl)  [unwired: 2 in, 2 out]
        n70 = property on="Position.Axis 1::15" class="DigNum (strict)"() -> ("Value"=w189:dbl)  [unwired: 2 in, 2 out]
        n71 = property on="value9::19" class="DigNum (strict)"() -> ("Value"=w190:dbl)  [unwired: 2 in, 2 out]
        n72 = call <vilib>:"Add State(s) to Queue__jki_lib_state_machine.vi"("State(s) in (\"\")"=w211) -> ("States Out"=w210:string)  [unwired: 14 in]
        n73 = Subtract(x=w182, y=w183) -> (x-y=w184:dbl)
        n74 = Subtract(x=w188, y=w187) -> (x-y=w185:dbl)
        n75 = Subtract(x=w189, y=w190) -> (x-y=w186:dbl)
        n76 = Multiply(x=-2, y=w186) -> (x*y=w193:dbl)
        n77 = Multiply(x=-2, y=w184) -> (x*y=w191:dbl)
        n78 = Multiply(x=-4, y=w185) -> (x*y=w194:dbl)
        n79 = Add(x=w191, y=w194) -> (x+y=w192:dbl)
        n80 = Add(x=w192, y=w193) -> (x+y=w195:dbl)
        n81 = Divide(x=w195, y=300) -> (x/y=w175:dbl)
        "Scatter Delay (ns)" <- w175
        n82 = property on="Position.Axis 3::6" class="DigNum (strict)"() -> ("Value"=w204:dbl)  [unwired: 2 in, 2 out]
        n83 = property on="value6::19" class="DigNum (strict)"() -> ("Value"=w207:dbl)  [unwired: 2 in, 2 out]
        n84 = property on="value5::19" class="DigNum (strict)"() -> ("Value"=w205:dbl)  [unwired: 2 in, 2 out]
        n85 = property on="position::23" class="DigNum (strict)"() -> ("Value"=w206:dbl)  [unwired: 2 in, 2 out]
        n86 = Subtract(x=w204, y=w205) -> (x-y=w199:dbl)
        n87 = Subtract(x=w206, y=w207) -> (x-y=w200:dbl)
        n88 = Multiply(x=-2, y=w199) -> (x*y=w201:dbl)
        n89 = Multiply(x=-4, y=w200) -> (x*y=w202:dbl)
        n90 = Add(x=w201, y=w202) -> (x+y=w203:dbl)
        n91 = Divide(x=w203, y=300) -> (x/y=w176:dbl)
        "Probe Delay (ns)" <- w176
        n92 = Subtract(x=w176, y=w175) -> (x-y=→"ProbeToScatter (ns)":dbl)
      }
      frame "Macro: Initialize" {
        w212 = "Data: Initialize\nInitialize Core Data\nUI: Initialize\nUI: Front Panel State >> Open"  # Data: Initialize Initialize Core Data UI: Initialize UI: Front Panel State >> Open
        # "Initialization Macro\n(This is called once, when the VI starts)"
        n93 = call <vilib>:"Add State(s) to Queue__jki_lib_state_machine.vi"("State(s) in Front (\"\")"=w212, "State(s) in (\"\")"=w216) -> ("States Out"=w215:string)  [unwired: 13 in]
      }
      frame "Macro: Exit" {
        # "Exit Macro\n(This is called once, when the VI exits)"
        n94 = Unbundle By Name(w223) -> ("Core.Close Panel on Exit?"=w222:bool)
        n95 = Select(t="UI: Front Panel State >> Close", s=w222, f="") -> (s? t:f=w219:string)
        n96 = call <vilib>:"Add State(s) to Queue__jki_lib_state_machine.vi"("State(s) in (\"\")"=w219, "State(s) at Back (\"\")"="Data: Cleanup\nExit") -> ("States Out"=w217:string)  [unwired: 13 in]
        n97 = call <vilib>:"Add State(s) to Queue__jki_lib_state_machine.vi"("State(s) in Front (\"\")"=w217, "State(s) in (\"\")"=w226) -> ("States Out"=w225:string)  [unwired: 13 in]
      }
      frame "---------- New Category ----------" {
        # "Template Separator\n(You can make a copy of, or modify, this frame)"
        n98 = call <vilib>:"Add State(s) to Queue__jki_lib_state_machine.vi"("State(s) in (\"\")"=w230) -> ("States Out"=w229:string)  [unwired: 14 in]
      }
      frame "Action: Fire" {
        # "Your code here.\n(You can make a copy of, or modify, this frame)"
        n99 = property on="fire::10" class="Str"(error in=w232, "Val(Sgnl)"="fire>>force" ("Value (Signaling)")) -> (error out=w231:errorcluster)  [unwired: 1 in, 1 out]
        n100 = call <vilib>:"Add State(s) to Queue__jki_lib_state_machine.vi"("State(s) in (\"\")"=w236) -> ("States Out"=w235:string)  [unwired: 14 in]
      }
    }
  }
